vi "Update Servo Parameters.vi"(8 "error in":errorcluster, 11 "tCRD in":refnum<class "Open Path CRD.lvclass">) -> (0 "error out":errorcluster, 3 "tCRD out":refnum<class "Open Path CRD.lvclass">)   [LabVIEW 2015, in "Open Path CRD.lvclass"]
uses:
  Open Path CRD.lvclass
  Open Path CRD.lvclass/Open Path CRD.ctl
  Reusable/Instrument/Instrument.lvclass/Instrument.ctl
  Switch/Servo Switch.lvclass/Servo Switch.ctl
  Accessors/Read Servo Switch.vi
  Reusable/Instrument/Read Log Session.vi
  Switch/Servo Switch.lvclass
  <userlib>/_Session Fwk/Session - Root.lvclass
  Reusable/Switch/Switch.lvclass
  Reusable/Session Log/System Log.lvclass
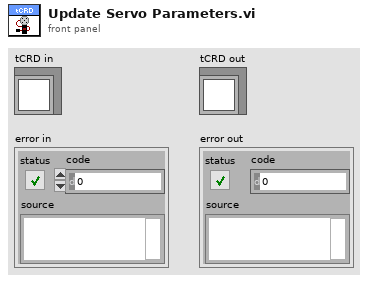
[diagram p1: front panel]
types:
  T1 = typedef "Session - Root.lvclass/Session Handle.ctl" = refnum<data-value>
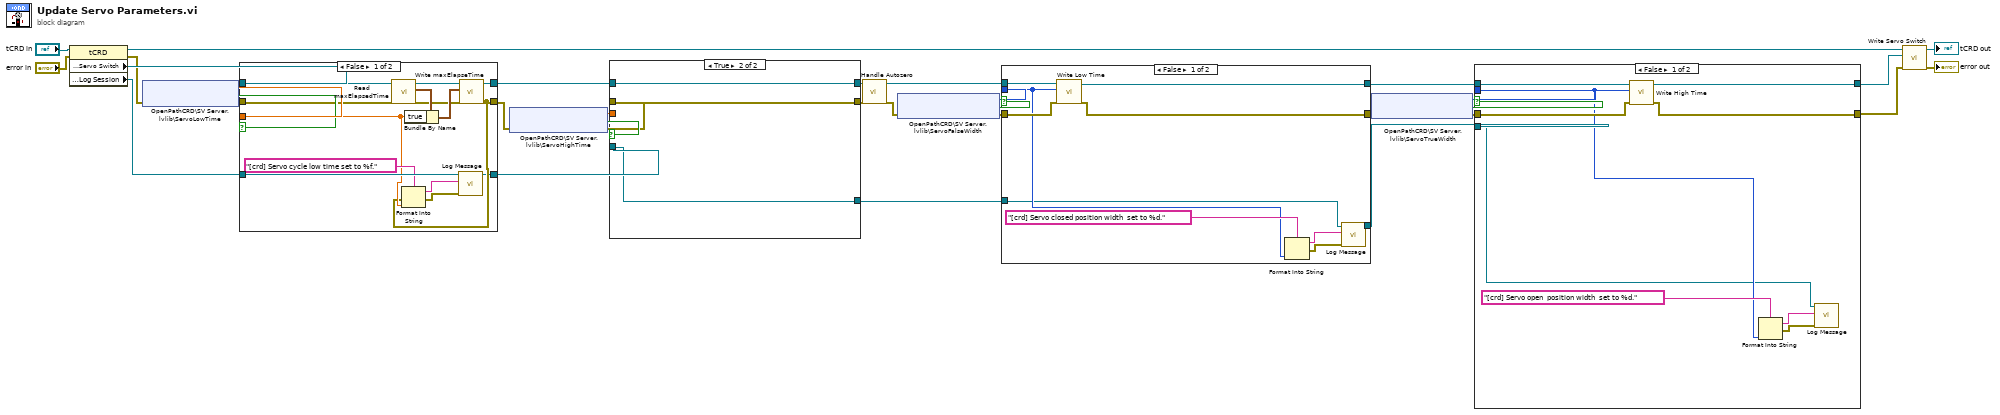
[diagram p0: block diagram]
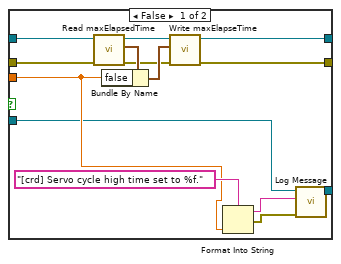
[diagram p4: hidden frame]
diagram:
  n1 = property class="tCRD"(reference="tCRD in", error in="error in") -> (reference out=w8:refnum<class "Open Path CRD.lvclass">, error out=w5:errorcluster, "Accessors:Servo Switch"=w7:refnum<class "Servo Switch.lvclass">, "Accessors:Log Session"=w4:T1)
  n2 = shared-variable "OpenPathCRD\\SV Server.lvlib\\ServoLowTime"(error in=w5) -> (w21:sgl, error out=w15:errorcluster, w20:bool)  [unwired: 1 in]
  n3 = case shown="False" w20 {
    tunnel: w15 -> [w43 w50]
    tunnel: [w41 w49] -> w22
    tunnel: w21 -> [w38 _]
    tunnel: w7 -> [w47 w49]
    tunnel: [w37 w50] -> w14
    tunnel: w4 -> [w40 w48]
    tunnel: [w34 w48] -> w3
    frame False {
      n4 = call "Read maxElapsedTime.vi"("error in"=w43, "Switch in"=w47) -> ("error out"=w42:errorcluster, "maxElapsedTime"=w46:cluster{"true":sgl, "false":sgl}, "Switch out"=w45:refnum<class "Servo Switch.lvclass">)  [unwired: 7 in]
      n5 = Bundle By Name(cluster=w46, "true"=w38) -> (w44:cluster{"true":sgl, "false":sgl})
      n6 = call "Write maxElapseTime.vi"("error in"=w42, "maxElapsedTime"=w44, "Switch in"=w45) -> ("error out"=w37:errorcluster, "Switch out"=w41:refnum<class "Servo Switch.lvclass">)  [unwired: 7 in]
      n7 = Format Into String(format string="[crd] Servo cycle low time set to %f.", error in=w37, w38) -> (resulting string=w35:string, error out=w36:errorcluster)  [unwired: 1 in]
      n8 = call "Log Message.vi"("error in"=w36, "MSG In"=w35, "session in"=w40) -> ("session out"=w34:T1)  [unwired: 7 in, 1 out]
    }
    frame True {
    }
  }
  n9 = shared-variable "OpenPathCRD\\SV Server.lvlib\\ServoHighTime"(error in=w14) -> (w23:sgl, error out=w13:errorcluster, w24:bool)  [unwired: 1 in]
  n10 = case shown="True" w24 {
    tunnel: w22 -> [w64 w67]
    tunnel: [w60 w67] -> w25
    tunnel: w23 -> [w53 _]
    tunnel: w13 -> [w63 w66]
    tunnel: [w57 w66] -> w12
    tunnel: w3 -> [w52 w65]
    tunnel: [w51 w65] -> w1
    frame False {
      n11 = call "Read maxElapsedTime.vi"("error in"=w63, "Switch in"=w64) -> ("error out"=w58:errorcluster, "maxElapsedTime"=w62:cluster{"true":sgl, "false":sgl}, "Switch out"=w59:refnum<class "Servo Switch.lvclass">)  [unwired: 7 in]
      n12 = Bundle By Name(cluster=w62, "false"=w53) -> (w61:cluster{"true":sgl, "false":sgl})
      n13 = call "Write maxElapseTime.vi"("error in"=w58, "maxElapsedTime"=w61, "Switch in"=w59) -> ("error out"=w57:errorcluster, "Switch out"=w60:refnum<class "Servo Switch.lvclass">)  [unwired: 7 in]
      n14 = Format Into String(format string="[crd] Servo cycle high time set to %f.", w53) -> (resulting string=w54:string, error out=w55:errorcluster)  [unwired: 2 in]
      n15 = call "Log Message.vi"("error in"=w55, "MSG In"=w54, "session in"=w52) -> ("session out"=w51:T1)  [unwired: 7 in, 1 out]
    }
    frame True {
    }
  }
  n16 = call "Handle Autozero.vi"("error in"=w12, "Servo Switch in"=w25) -> ("error out"=w32:errorcluster, "Servo Switch out"=w31:refnum<class "Servo Switch.lvclass">)  [unwired: 8 in]
  n17 = shared-variable "OpenPathCRD\\SV Server.lvlib\\ServoFalseWidth"(error in=w32) -> (w27:u32, error out=w33:errorcluster, w26:bool)  [unwired: 1 in]
  n18 = case shown="False" w26 {
    tunnel: w31 -> [w77 w80]
    tunnel: w27 -> [w70 _]
    tunnel: [w76 w80] -> w28
    tunnel: w33 -> [w75 w79]
    tunnel: [w74 w79] -> w11
    tunnel: [w69 w78] -> w2
    tunnel: w1 -> [w68 w78]
    frame False {
      n19 = call "Write Low Time.vi"("error in (no error)"=w75, "Low Time"=w70, "Servo Switch in"=w77) -> ("error out"=w74:errorcluster, "Servo Switch out"=w76:refnum<class "Servo Switch.lvclass">)  [unwired: 7 in]
      n20 = Format Into String(format string="[crd] Servo closed position width  set to %d.", w70) -> (resulting string=w71:string, error out=w72:errorcluster)  [unwired: 2 in]
      n21 = call "Log Message.vi"("error in"=w72, "MSG In"=w71, "session in"=w68) -> ("session out"=w69:T1)  [unwired: 7 in, 1 out]
    }
    frame True {
    }
  }
  n22 = shared-variable "OpenPathCRD\\SV Server.lvlib\\ServoTrueWidth"(error in=w11) -> (w30:u32, error out=w10:errorcluster, w29:bool)  [unwired: 1 in]
  n23 = case shown="False" w29 {
    tunnel: w28 -> [w89 w91]
    tunnel: [w88 w91] -> w19
    tunnel: w30 -> [w82 _]
    tunnel: w10 -> [w87 w90]
    tunnel: [w86 w90] -> w18
    tunnel: w2 -> [w81 _]
    frame False {
      n24 = call "Write High Time.vi"("error in (no error)"=w87, "High Time"=w82, "Servo Switch in"=w89) -> ("error out"=w86:errorcluster, "Servo Switch out"=w88:refnum<class "Servo Switch.lvclass">)  [unwired: 7 in]
      n25 = Format Into String(format string="[crd] Servo open  position width  set to %d.", w82) -> (resulting string=w83:string, error out=w84:errorcluster)  [unwired: 2 in]
      n26 = call "Log Message.vi"("error in"=w84, "MSG In"=w83, "session in"=w81) -> ()  [unwired: 7 in, 2 out]
    }
    frame True {
    }
  }
  n27 = call "Write Servo Switch.vi"("error in (no error)"=w18, "Servo Switch"=w19, "tCRD in"=w8) -> ("error out"=→"error out":errorcluster, "tCRD out"=→"tCRD out":refnum<class "Open Path CRD.lvclass">)  [unwired: 7 in]
